vi "Create Event.vi"(8 "error in (no error)":errorcluster, 11 "TAS_Event.lvclass":refnum<class "TAS_Event.lvclass">) -> (0 "error out":errorcluster, 3 "TAS Event Out":refnum<user-event>)   [LabVIEW 2012, in "TAS_Event.lvclass"]
uses:
  TAS_Event.lvclass
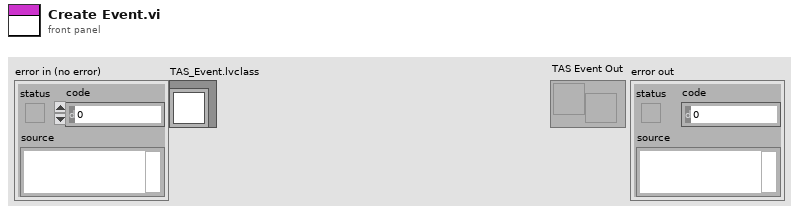
[diagram p1: front panel]
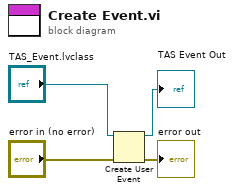
[diagram p0: block diagram]
diagram:
  n1 = Create User Event(user event datatype="TAS_Event.lvclass", error in="error in (no error)") -> (user event=→"TAS Event Out":refnum<user-event>, error out=→"error out":errorcluster)
